vi "Exercises_4-9.vi"() -> ()   [LabVIEW 2014]
panel:
  in  "Max Wind Speed":dbl
  in  "Current Wind Speed":dbl
  out "Warning?":bool
  out "Warning Text":string
  in  "Min Temp":dbl
  in  "Max Temp":dbl
  in  "Current Temp":dbl
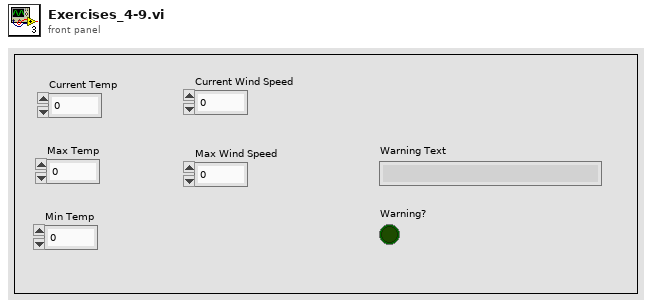
[diagram p1: front panel]
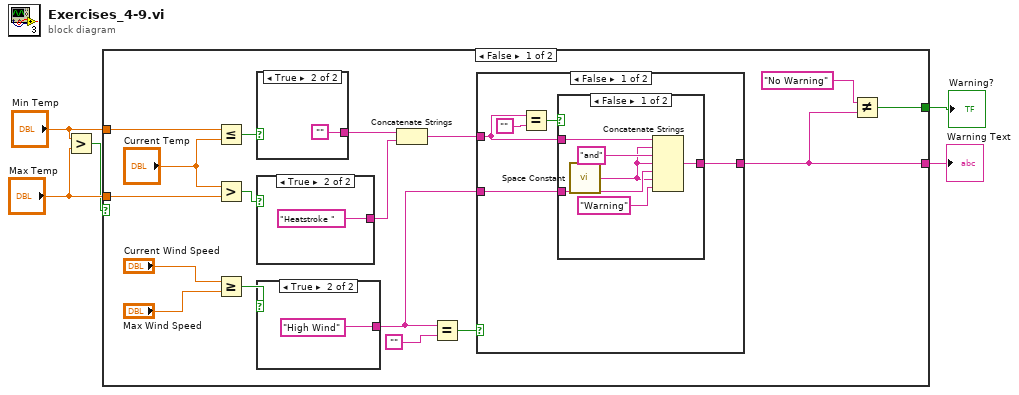
[diagram p0: block diagram]
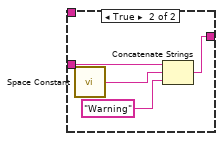
[diagram p2: hidden frame]
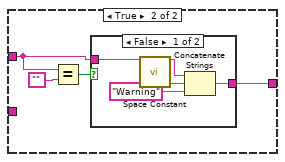
[diagram p3: hidden frame]
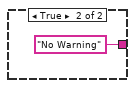
[diagram p4: hidden frame]
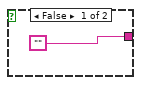
[diagram p5: hidden frame]
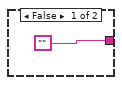
[diagram p6: hidden frame]
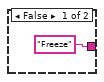
[diagram p7: hidden frame]
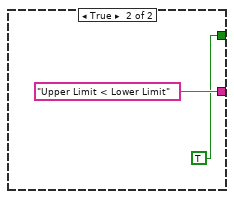
[diagram p8: hidden frame]
diagram:
  n1 = Greater?(x="Min Temp", y="Max Temp") -> (0:w1:bool)
  n2 = case shown="False" w1 {
    tunnel: [w9 "Upper Limit < Lower Limit"] -> w5
    tunnel: [w22 TRUE] -> w4
    tunnel: "Min Temp" -> [w21 _]
    tunnel: "Max Temp" -> [w19 _]
    frame False {
      n3 = Less Or Equal?(x=w21, y="Current Temp") -> (x <= y?=w18:bool)
      n4 = Greater?(x="Current Temp", y=w19) -> (0:w17:bool)
      n5 = Greater Or Equal?(x="Current Wind Speed", y="Max Wind Speed") -> (x >= y?=w13:bool)
      n6 = case shown="True" w18 {
        tunnel: ["Freeze" ""] -> w15
        frame False {
        }
        frame True {
        }
      }
      n7 = case shown="True" w17 {
        tunnel: ["" "Heatstroke "] -> w16
        frame False {
        }
        frame True {
        }
      }
      n8 = case shown="True" w13 {
        tunnel: ["" "High Wind"] -> w7
        frame False {
        }
        frame True {
        }
      }
      n9 = Concatenate Strings(w15, w16) -> (w11:string)
      n10 = Equal?(x=w7, y="") -> (x = y?=w8:bool)
      n11 = case shown="False" w8 {
        tunnel: w11 -> [w25 w39]
        tunnel: [w23 w38] -> w9
        tunnel: w7 -> [w24 _]
        frame False {
          n12 = Equal?(x=w25, y="") -> (x = y?=w27:bool)
          n13 = case shown="False" w27 {
            tunnel: w25 -> [w33 _]
            tunnel: [w32 w34] -> w23
            tunnel: w24 -> [w30 w37]
            frame False {
              n14 = call <vilib>:"Space Constant.vi"() -> ("String"=w29:string)
              n15 = Concatenate Strings(w33, w29, "and", w29, w30, w29, "Warning") -> (w32:string)
            }
            frame True {
              n16 = call <vilib>:"Space Constant.vi"() -> ("String"=w36:string)
              n17 = Concatenate Strings(w37, w36, "Warning") -> (w34:string)
            }
          }
        }
        frame True {
          n18 = Equal?(x=w39, y="") -> (x = y?=w40:bool)
          n19 = case shown="False" w40 {
            tunnel: w39 -> [w43 _]
            tunnel: [w42 "No Warning"] -> w38
            frame False {
              n20 = call <vilib>:"Space Constant.vi"() -> ("String"=w45:string)
              n21 = Concatenate Strings(w43, w45, "Warning") -> (w42:string)
            }
            frame True {
            }
          }
        }
      }
      n22 = Not Equal?(x="No Warning", y=w9) -> (x != y?=w22:bool)
    }
    frame True {
    }
  }
  "Warning Text" <- w5
  "Warning?" <- w4
